vi "Test MQTT_Client API.vi"() -> ()   [LabVIEW 2020]
doc: "MQTT_Client API Tester."
uses:
  MQTT_Client.lvlib
panel:
  out "Connected":bool
  in  "Topic":string
  in  "Subscribe to topic":bool
  in  "Disconnect Client":bool
  in  "IP Address":string="localhost"
  in  "Remote Port":u16=1883
  in  "Connect Client":bool
  in  "Run as Singleton?":bool
  in  "Show Block Diagram":bool
  in  "Refresh Modules":bool
  out "Active Modules":string[](array[string])
  in  "Stop Module":bool
  in  "Select Module":i32(ring)=-1 caption="Select Module\nTo send Request to" items=["All"=-1]
  in  "Run New Module":bool
  in  "Hide Module Panel":bool
  in  "Show Module Panel":bool
  out "Status":string
  # "This VI tests the API for the Module."
  # "This is a DQMH Cloneable Module\nIt can be connected to an MQTT Broker\n1. Go to the virtual Folder called 'MQTT Local Broker'\n2. Run the 'Simple MQTT Broker.vi'\n3. Run The API Tester an Connect to the IP and PORT of the MQTT Broker\n4. Add in the Broker Secction or your Panther Sniffer for DQMH the MQTT Broker\n5. Add a the DQMH Module to the Modules Section of your app\n6. Tap your Module on the app and you'll se all the Status Updated Broadcast\n\n\nPanther Sniffer for DQMH(r) available on \nGoogle Play Store.\nhttps://play.google.com/store/apps/details?id=mx.com.pantherlab.pantherSniffer"
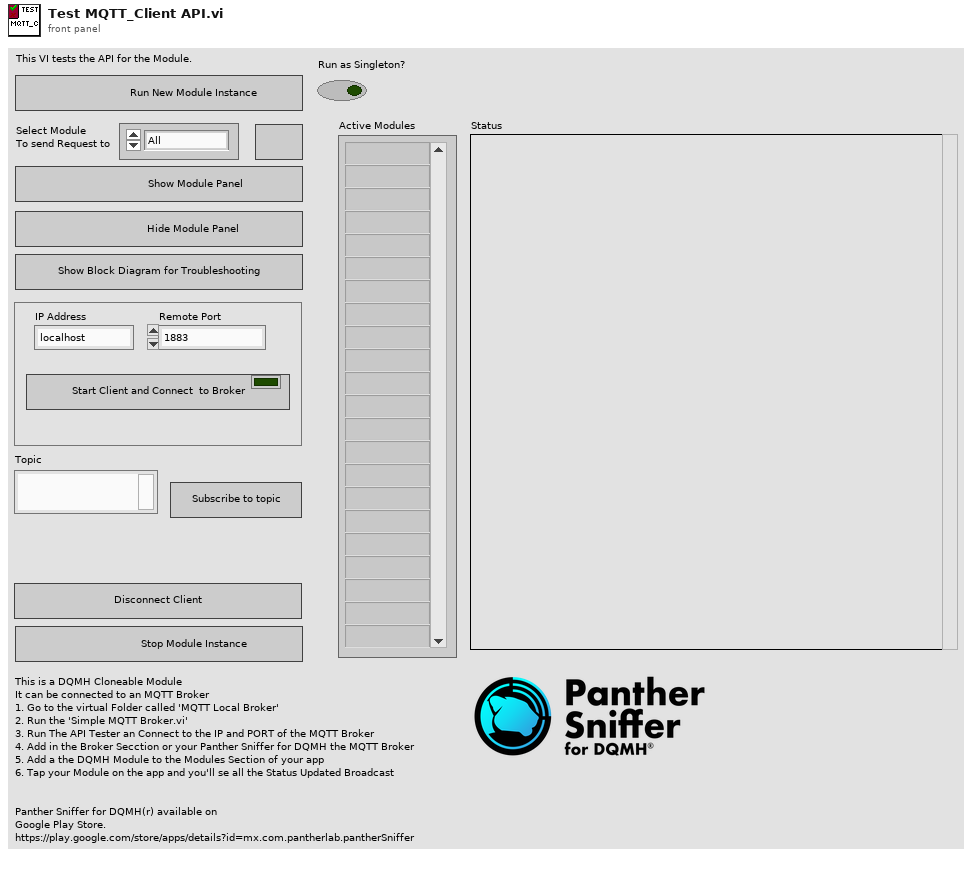
[diagram p1: front panel]
types:
  T1 = typedef "MQTT_Client.lvlib/Broadcast Events--cluster.ctl" = cluster{"Module Did Init":refnum<user-event>, "Status Updated":refnum<user-event>, "Error Reported":refnum<user-event>, "Module Did Stop":refnum<user-event>, "Update Module Execution Status":refnum<user-event>, "Client Status":refnum<user-event>}
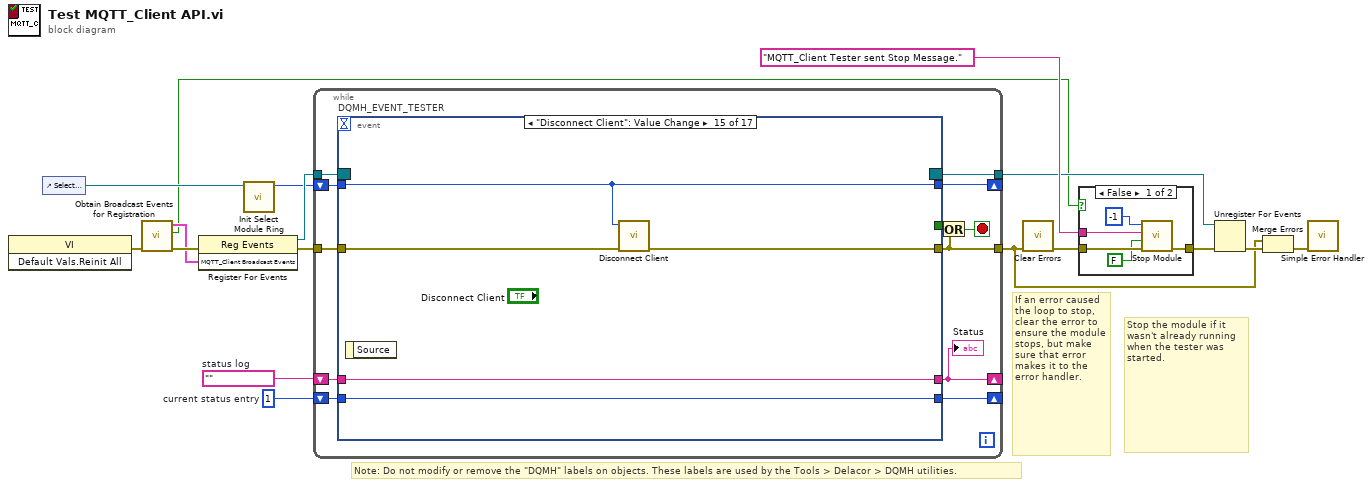
[diagram p0: block diagram]
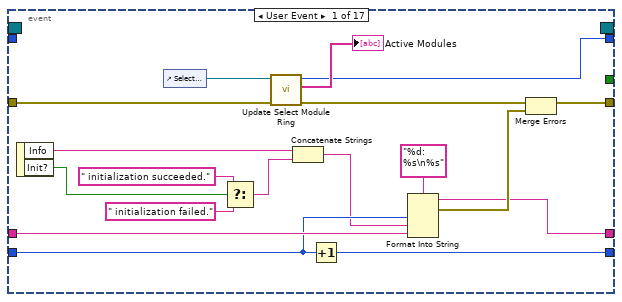
[diagram p3: hidden frame]
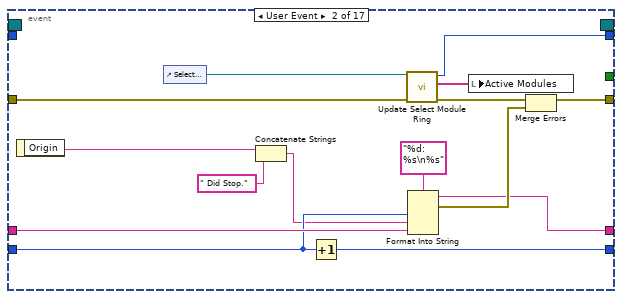
[diagram p4: hidden frame]
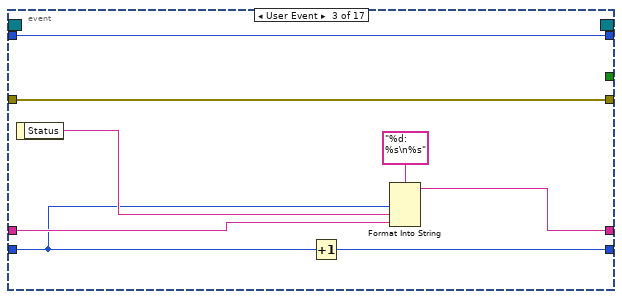
[diagram p5: hidden frame]
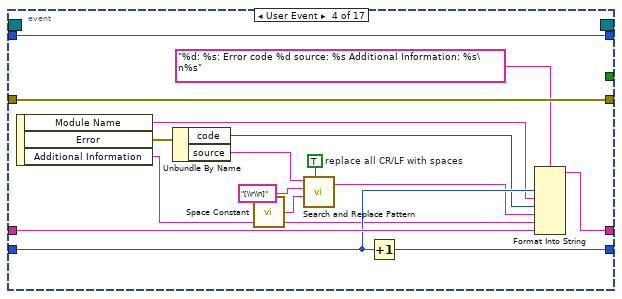
[diagram p6: hidden frame]
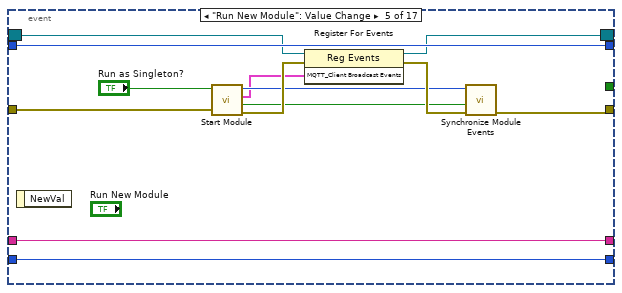
[diagram p7: hidden frame]
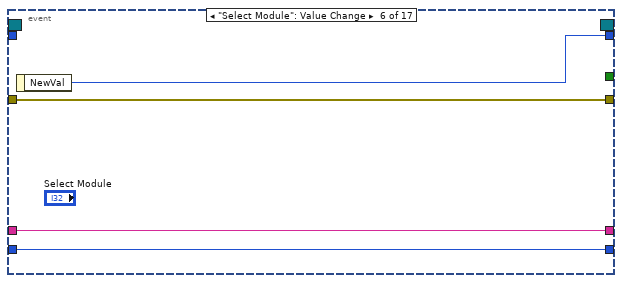
[diagram p8: hidden frame]
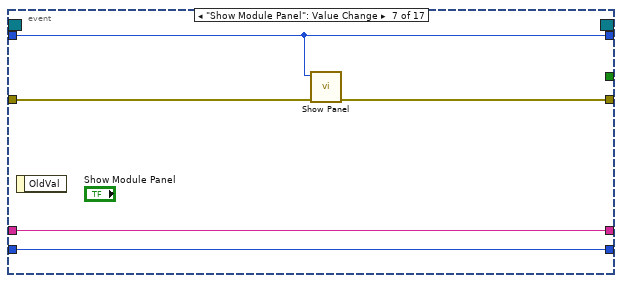
[diagram p9: hidden frame]
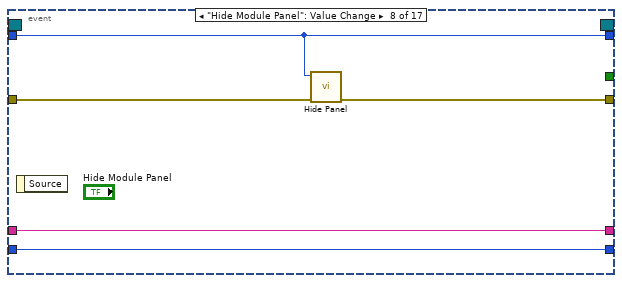
[diagram p10: hidden frame]
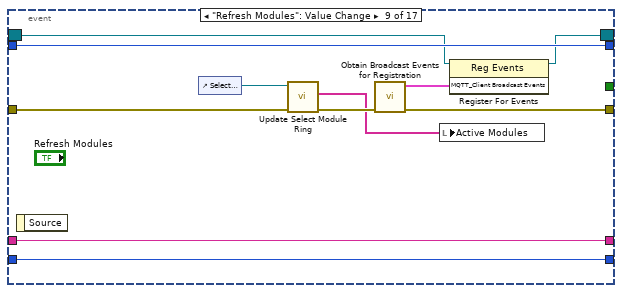
[diagram p11: hidden frame]
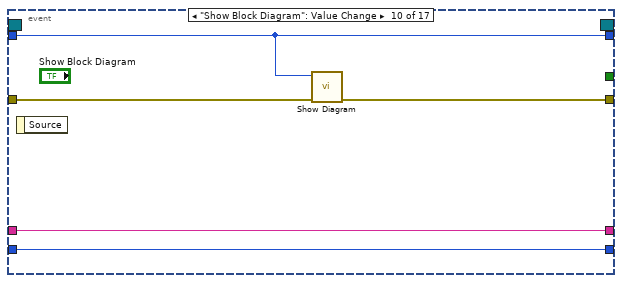
[diagram p12: hidden frame]
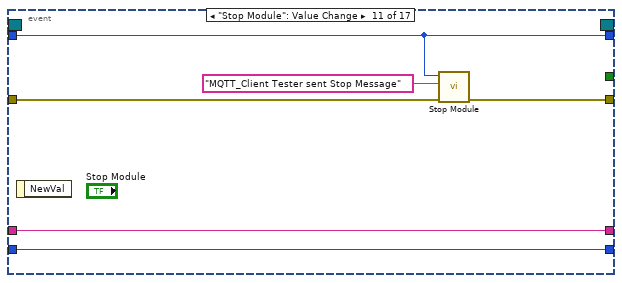
[diagram p13: hidden frame]
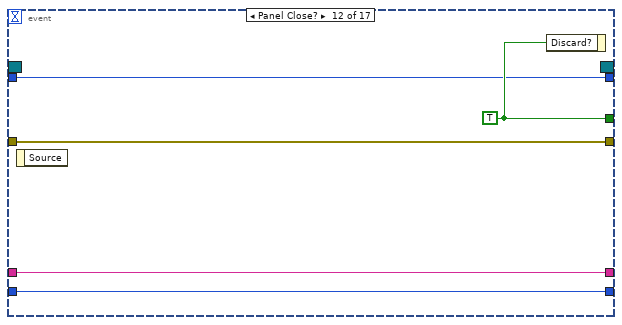
[diagram p14: hidden frame]
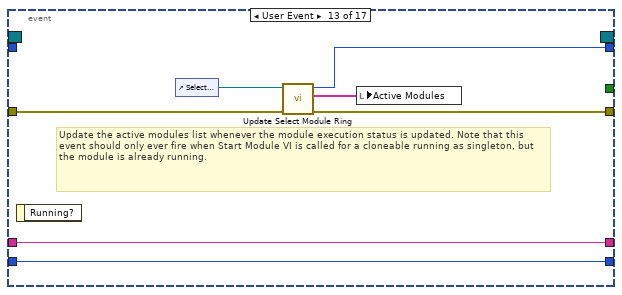
[diagram p15: hidden frame]
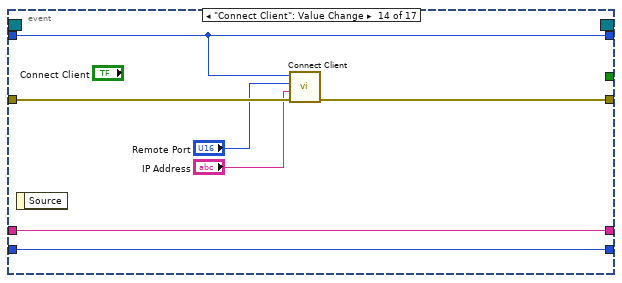
[diagram p16: hidden frame]
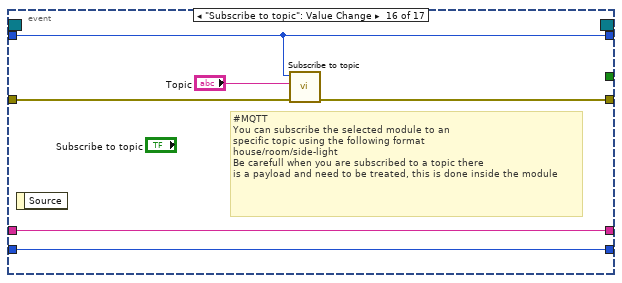
[diagram p17: hidden frame]
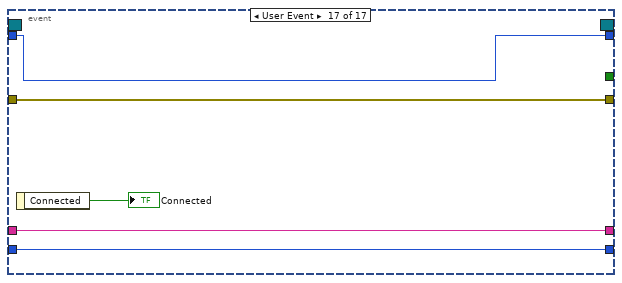
[diagram p18: hidden frame]
diagram:
  w7 = 1  # current status entry
  w8 = ""  # status log
  # "Stop the module if it wasn't already running when the tester was started."
  # "If an error caused the loop to stop, clear the error to ensure the module stops, but make sure that error makes it to the error handler."
  # "Note: Do not modify or remove the \"DQMH\" labels on objects. These labels are used by the Tools > Delacor > DQMH utilities."
  n1 = invoke class="VI" method="Default Vals.Reinit All"() -> (error out=w11:errorcluster)  [unwired: 3 in, 2 out]
  n2 = control-ref of="Select Module"() -> (w5:refnum<vi>)
  n3 = call "Obtain Broadcast Events for Registration.vi"("error in (no error)"=w11) -> ("error out"=w10:errorcluster, "Already running?"=w1:bool, "MQTT_Client Broadcast Events"=w4:T1)  [unwired: 8 in]
  n4 = register-events(error in=w10, w4) -> (reference out=w9:refnum<event-registration>, error out=w15:errorcluster)  [unwired: 1 in]
  n5 = call "Init Select Module Ring.vi"("Select Module Ring Ref"=w5) -> ("Value for All Modules"=w6:i32)  [unwired: 8 in, 2 out]
  n6 = while {
    tunnel: w9 -> [w27]
    tunnel: [w28] -> w12
    tunnel: w15 -> [w29]
    shift-right: [w22] -> _
    shift-left: w8 -> [w24]
    shift-right: [w23] -> _
    shift-left: w7 -> [w25]
    shift-right: [w19] -> _
    shift-left: w6 -> [w20]
    tunnel: [w18] -> w2
    stop <- w21 stop-if-true
    n7 = event "DQMH_EVENT_TESTER" shown="[14] \"Disconnect Client\": Value Change" {
      selector: w27 -> [_ _ _ _ w92 _ _ _ w117 _ _ _ _ _ _ _ _]
      dyn-events: [_ _ _ _ w91 _ _ _ w116 _ _ _ _ _ _ _ _] -> w18
      timeout: _ -> [_ _ _ _ _ _ _ _ _ _ _ _ _ _ _ _ _]
      tunnel: [_ _ _ _ _ _ _ _ _ _ _ w139 _ _ _ _ _] -> w26
      tunnel: [w44 w59 w70 w86 w96 w103 w107 w112 w122 w128 w134 w140 w146 w153 w158 w164 w170] -> w28
      tunnel: w29 -> [w46 w61 w70 w86 w97 w103 w108 w113 w124 w129 w135 w140 w147 w154 w159 w165 w170]
      tunnel: w25 -> [w41 w56 w63 w80 w94 w101 w105 w110 w120 w126 w132 w137 w144 w151 w156 w162 w167]
      tunnel: w24 -> [w42 w57 w66 w82 w95 w102 w106 w111 w121 w127 w133 w138 w145 w152 w157 w163 w168]
      tunnel: [w39 w54 w67 w77 w95 w102 w106 w111 w121 w127 w133 w138 w145 w152 w157 w163 w168] -> w22
      tunnel: [w40 w55 w69 w83 w94 w101 w105 w110 w120 w126 w132 w137 w144 w151 w156 w162 w167] -> w23
      tunnel: w20 -> [_ _ w64 w84 w93 _ w104 w109 w119 w125 w131 w136 _ w150 w155 w161 w169]
      tunnel: [w34 w51 w64 w84 w93 w100 w104 w109 w119 w125 w131 w136 w142 w150 w155 w161 w169] -> w19
      event User Event {
        n8 = event-data() -> ("Info"=w38:string, "Init?"=w31:bool)  [unwired: 1 in]
        n9 = control-ref of="Select Module"() -> (w36:refnum<vi>)
        n10 = Select(t=" initialization succeeded.", s=w31, f=" initialization failed.") -> (s? t:f=w30:string)
        n11 = call "Update Select Module Ring.vi"("error in (no error)"=w46, "Select Module Ring Ref"=w36) -> ("error out"=w45:errorcluster, "Active Modules (Array)"=→"Active Modules":string[], "New Module Ring Value"=w34:i32)  [unwired: 7 in]
        n12 = Concatenate Strings(w38, w30) -> (w37:string)
        n13 = Increment(x=w41) -> (x+1=w40:i32)
        n14 = Format Into String(format string="%d: %s\n%s", w41, w37, w42) -> (resulting string=w39:string, error out=w47:errorcluster)  [unwired: 2 in]
        n15 = Merge Errors(w45, w47) -> (w44:errorcluster)
      }
      event User Event {
        n16 = event-data() -> ("Origin"=w49:string)  [unwired: 1 in]
        n17 = control-ref of="Select Module"() -> (w53:refnum<vi>)
        n18 = Concatenate Strings(w49, " Did Stop.") -> (w48:string)
        n19 = Increment(x=w56) -> (x+1=w55:i32)
        n20 = call "Update Select Module Ring.vi"("error in (no error)"=w61, "Select Module Ring Ref"=w53) -> ("error out"=w60:errorcluster, "Active Modules (Array)"=w52:string[], "New Module Ring Value"=w51:i32)  [unwired: 7 in]
        n21 = Format Into String(format string="%d: %s\n%s", w56, w48, w57) -> (resulting string=w54:string, error out=w62:errorcluster)  [unwired: 2 in]
        n22 = local write "Active Modules"(w52) -> ()
        n23 = Merge Errors(w60, w62) -> (w59:errorcluster)
      }
      event User Event {
        n24 = event-data() -> ("Status"=w65:string)  [unwired: 1 in]
        n25 = Increment(x=w63) -> (x+1=w69:i32)
        n26 = Format Into String(format string="%d: %s\n%s", w63, w65, w66) -> (resulting string=w67:string)  [unwired: 2 in, 1 out]
      }
      event User Event {
        w78 = TRUE  # replace all CR/LF with spaces
        n27 = event-data() -> ("Module Name"=w73:string, "Error"=w85:errorcluster, "Additional Information"=w71:string)  [unwired: 1 in]
        n28 = Unbundle By Name(w85) -> ("code"=w74:i32, "source"=w75:string)
        n29 = call <vilib>:"Space Constant.vi"() -> ("String"=w79:string)
        n30 = call <vilib>:"Search and Replace Pattern.vi"("string"=w75, "regular expression (\"\")"="[\\r\\n]" ("regular expression (\"\")"), "replace string (\"\")"=w79, "replace all? (F)"=w78) -> ("result string"=w76:string)  [unwired: 1 in, 1 out]
        n31 = Increment(x=w80) -> (x+1=w83:i32)
        n32 = Format Into String(format string="%d: %s: Error code %d source: %s Additional Information: %s\n%s", w80, w73, w74, w76, w71, w82) -> (resulting string=w77:string)  [unwired: 2 in, 1 out]
      }
      event "Run New Module": Value Change {
        n33 = event-data() -> ()  [unwired: 1 in, 1 out]
        n34 = call "Start Module.vi"("error in (no error)"=w97, "Run as Singleton? (F)"="Run as Singleton?") -> ("error out"=w98:errorcluster, "Wait for Event Sync?"=w89:bool, "MQTT_Client Broadcast Events"=w88:T1, "Module ID"=w90:i32)  [unwired: 6 in]
        n35 = register-events(reference=w92, error in=w98, w88) -> (reference out=w91:refnum<event-registration>, error out=w99:errorcluster)
        n36 = call "Synchronize Module Events.vi"("error in (no error)"=w99, "Wait for Event Sync?"=w89, "Module ID"=w90) -> ("error out"=w96:errorcluster)  [unwired: 7 in, 1 out]
      }
      event "Select Module": Value Change {
        n37 = event-data() -> ("NewVal"=w100:i32)  [unwired: 1 in]
      }
      event "Show Module Panel": Value Change {
        n38 = event-data() -> ()  [unwired: 1 in, 1 out]
        n39 = call "Show Panel.vi"("error in (no error)"=w108, "Module ID"=w104) -> ("error out"=w107:errorcluster)  [unwired: 9 in]
      }
      event "Hide Module Panel": Value Change {
        n40 = event-data() -> ()  [unwired: 1 in, 1 out]
        n41 = call "Hide Panel.vi"("error in (no error)"=w113, "Module ID"=w109) -> ("error out"=w112:errorcluster)  [unwired: 9 in]
      }
      event "Refresh Modules": Value Change {
        n42 = event-data() -> ()  [unwired: 1 in, 1 out]
        n43 = control-ref of="Select Module"() -> (w118:refnum<vi>)
        n44 = call "Update Select Module Ring.vi"("error in (no error)"=w124, "Select Module Ring Ref"=w118) -> ("error out"=w123:errorcluster, "Active Modules (Array)"=w114:string[])  [unwired: 7 in, 1 out]
        n45 = call "Obtain Broadcast Events for Registration.vi"("error in (no error)"=w123) -> ("error out"=w122:errorcluster, "MQTT_Client Broadcast Events"=w115:T1)  [unwired: 8 in, 1 out]
        n46 = local write "Active Modules"(w114) -> ()
        n47 = register-events(reference=w117, w115) -> (reference out=w116:refnum<event-registration>)  [unwired: 1 in, 1 out]
      }
      event "Show Block Diagram": Value Change {
        n48 = event-data() -> ()  [unwired: 1 in, 1 out]
        n49 = call "Show Diagram.vi"("error in (no error)"=w129, "Module ID"=w125) -> ("error out"=w128:errorcluster)  [unwired: 9 in]
      }
      event "Stop Module": Value Change {
        n50 = event-data() -> ()  [unwired: 1 in, 1 out]
        n51 = call "Stop Module.vi"("error in (no error)"=w135, "Origin"="MQTT_Client Tester sent Stop Message", "Module ID"=w131) -> ("error out"=w134:errorcluster)  [unwired: 8 in]
      }
      event Panel Close? {
        w139 = TRUE ("Discard?")
        n52 = event-data() -> ()  [unwired: 1 in, 1 out]
        n53 = event-data("Discard?"=w139) -> ()  [unwired: 1 in, 1 out]
      }
      event User Event {
        # "Update the active modules list whenever the module execution status is updated. Note that this event should only ever fire when Start Module VI is called for a cloneable running as singleton, but the module is already running."
        n54 = event-data() -> ()  [unwired: 1 in, 1 out]
        n55 = control-ref of="Select Module"() -> (w143:refnum<vi>)
        n56 = call "Update Select Module Ring.vi"("error in (no error)"=w147, "Select Module Ring Ref"=w143) -> ("error out"=w146:errorcluster, "Active Modules (Array)"=w141:string[], "New Module Ring Value"=w142:i32)  [unwired: 7 in]
        n57 = local write "Active Modules"(w141) -> ()
      }
      event "Connect Client": Value Change {
        n58 = event-data() -> ()  [unwired: 1 in, 1 out]
        n59 = call "Connect Client.vi"("error in (no error)"=w154, "IP Address"="IP Address", "Remote Port"="Remote Port", "Module ID"=w150) -> ("error out"=w153:errorcluster)  [unwired: 7 in]
      }
      event "Disconnect Client": Value Change {
        n60 = event-data() -> ()  [unwired: 1 in, 1 out]
        n61 = call "Disconnect Client.vi"("error in (no error)"=w159, "Module ID"=w155) -> ("error out"=w158:errorcluster)  [unwired: 9 in]
      }
      event "Subscribe to topic": Value Change {
        # "#MQTT   \nYou can subscribe the selected module to an \nspecific topic using the following format\nhouse/room/side-light\nBe carefull when you are subscribed to a topic there\nis a payload and need to be treated, this is done inside the module"
        n62 = event-data() -> ()  [unwired: 1 in, 1 out]
        n63 = call "Subscribe to topic.vi"("error in (no error)"=w165, "Topic"="Topic", "Module ID"=w161) -> ("error out"=w164:errorcluster)  [unwired: 8 in]
      }
      event User Event {
        n64 = event-data() -> ("Connected"=→"Connected":bool)  [unwired: 1 in]
      }
    }
    "Status" <- w22
    n65 = Or(x=w26, y=w28) -> (x .or. y?=w21:bool)
  }
  n66 = call <vilib>:"Clear Errors.vi"("error in (no error)"=w12) -> ("error out"=w14:errorcluster)  [unwired: 5 in, 1 out]
  n67 = case shown="False" w1 {
    tunnel: [w175 w176] -> w16
    tunnel: "MQTT_Client Tester sent Stop Message." ("Origin") -> [w173 _]
    tunnel: w14 -> [w174 w176]
    frame False {
      n68 = call "Stop Module.vi"("error in (no error)"=w174, "Wait for Module to stop? (F)"=FALSE ("Wait for Module to stop?"), "Origin"=w173, "Module ID"=-1 ("Stop all")) -> ("error out"=w175:errorcluster)  [unwired: 7 in]
    }
    frame True {
    }
  }
  n69 = Unregister For Events(event registration refnum=w2, error in=w16) -> (error out=w17:errorcluster)
  n70 = Merge Errors(w12, w17) -> (w13:errorcluster)
  n71 = call <vilib>:"Simple Error Handler.vi"("error in (no error)"=w13) -> ()  [unwired: 4 in, 5 out]
